vi "Create.vi"(8 "error in":errorcluster, 10 "Option String":string, 11 "Reset":bool) -> (0 "error out":errorcluster, 3 "Session Factory Out":refnum<class "Session Factory.lvclass">)   [LabVIEW 2020, in "IVI Scope Instrument.lvlib" / "Session Factory.lvclass"]
uses:
  Session Factory.lvclass
  Session Factory.lvclass/Session Factory.ctl
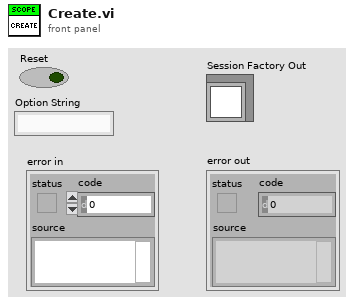
[diagram p1: front panel]
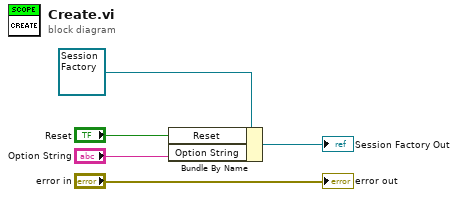
[diagram p0: block diagram]
diagram:
  n1 = Bundle By Name(cluster=refnum<class "Session Factory.lvclass"> refnum ("IVI Scope Instrument.lvlib:Session Factory.lvclass"), "Reset"="Reset", "Option String"="Option String") -> (→"Session Factory Out":refnum<class "Session Factory.lvclass">)
  "error out" <- "error in"
